vi "Force Sensing-Axial.vi"() -> ()   [LabVIEW 2010]
uses:
  <vilib>/Utility/file.llb/Write To Spreadsheet File (string).vi
panel:
  out "Shift 4":dbl
  out "Base 4":dbl format="%.3f"
  out "Channel 4":dbl format="%.2f"
  out "Calibration Constant":dbl
  in  "stop":bool
  in  "Force Scaling Factor":dbl=1.0
  in  "Record Switch":bool
  in  "file path (dialog if empty)":path=path "C:/Users/Berk/Desktop/closed_washer0_1"
  out "Measured Tip Forces [mN]":u8(slide) scale=0.0..10.0
  in  "Plot Switch":bool
  out "F [mN]":dbl format="%.1f"
  in  "sm130 IP Address":string="192.168.0.11"
  in  "Rebias":bool
  in  "Select Your Tool":T1(radio)
  out "Shift 3":dbl
  out "Shift 2":dbl
  out "Shift 1":dbl
  out "Channel 3":dbl format="%.2f"
  out "Channel 2":dbl format="%.2f"
  out "Channel 1":dbl format="%.2f"
  out "Base 3":dbl format="%.3f"
  out "Base 2":dbl format="%.3f"
  out "Base 1":dbl format="%.3f"
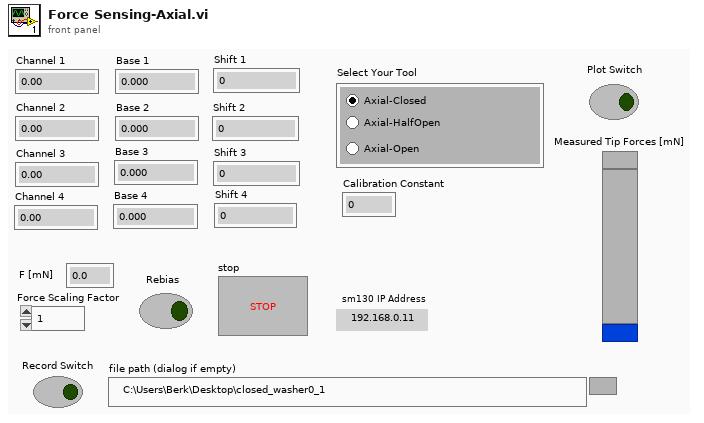
[diagram p1: front panel]
types:
  T1 = enum32{"Axial-Closed", "Axial-Open", "Axial-HalfOpen"}
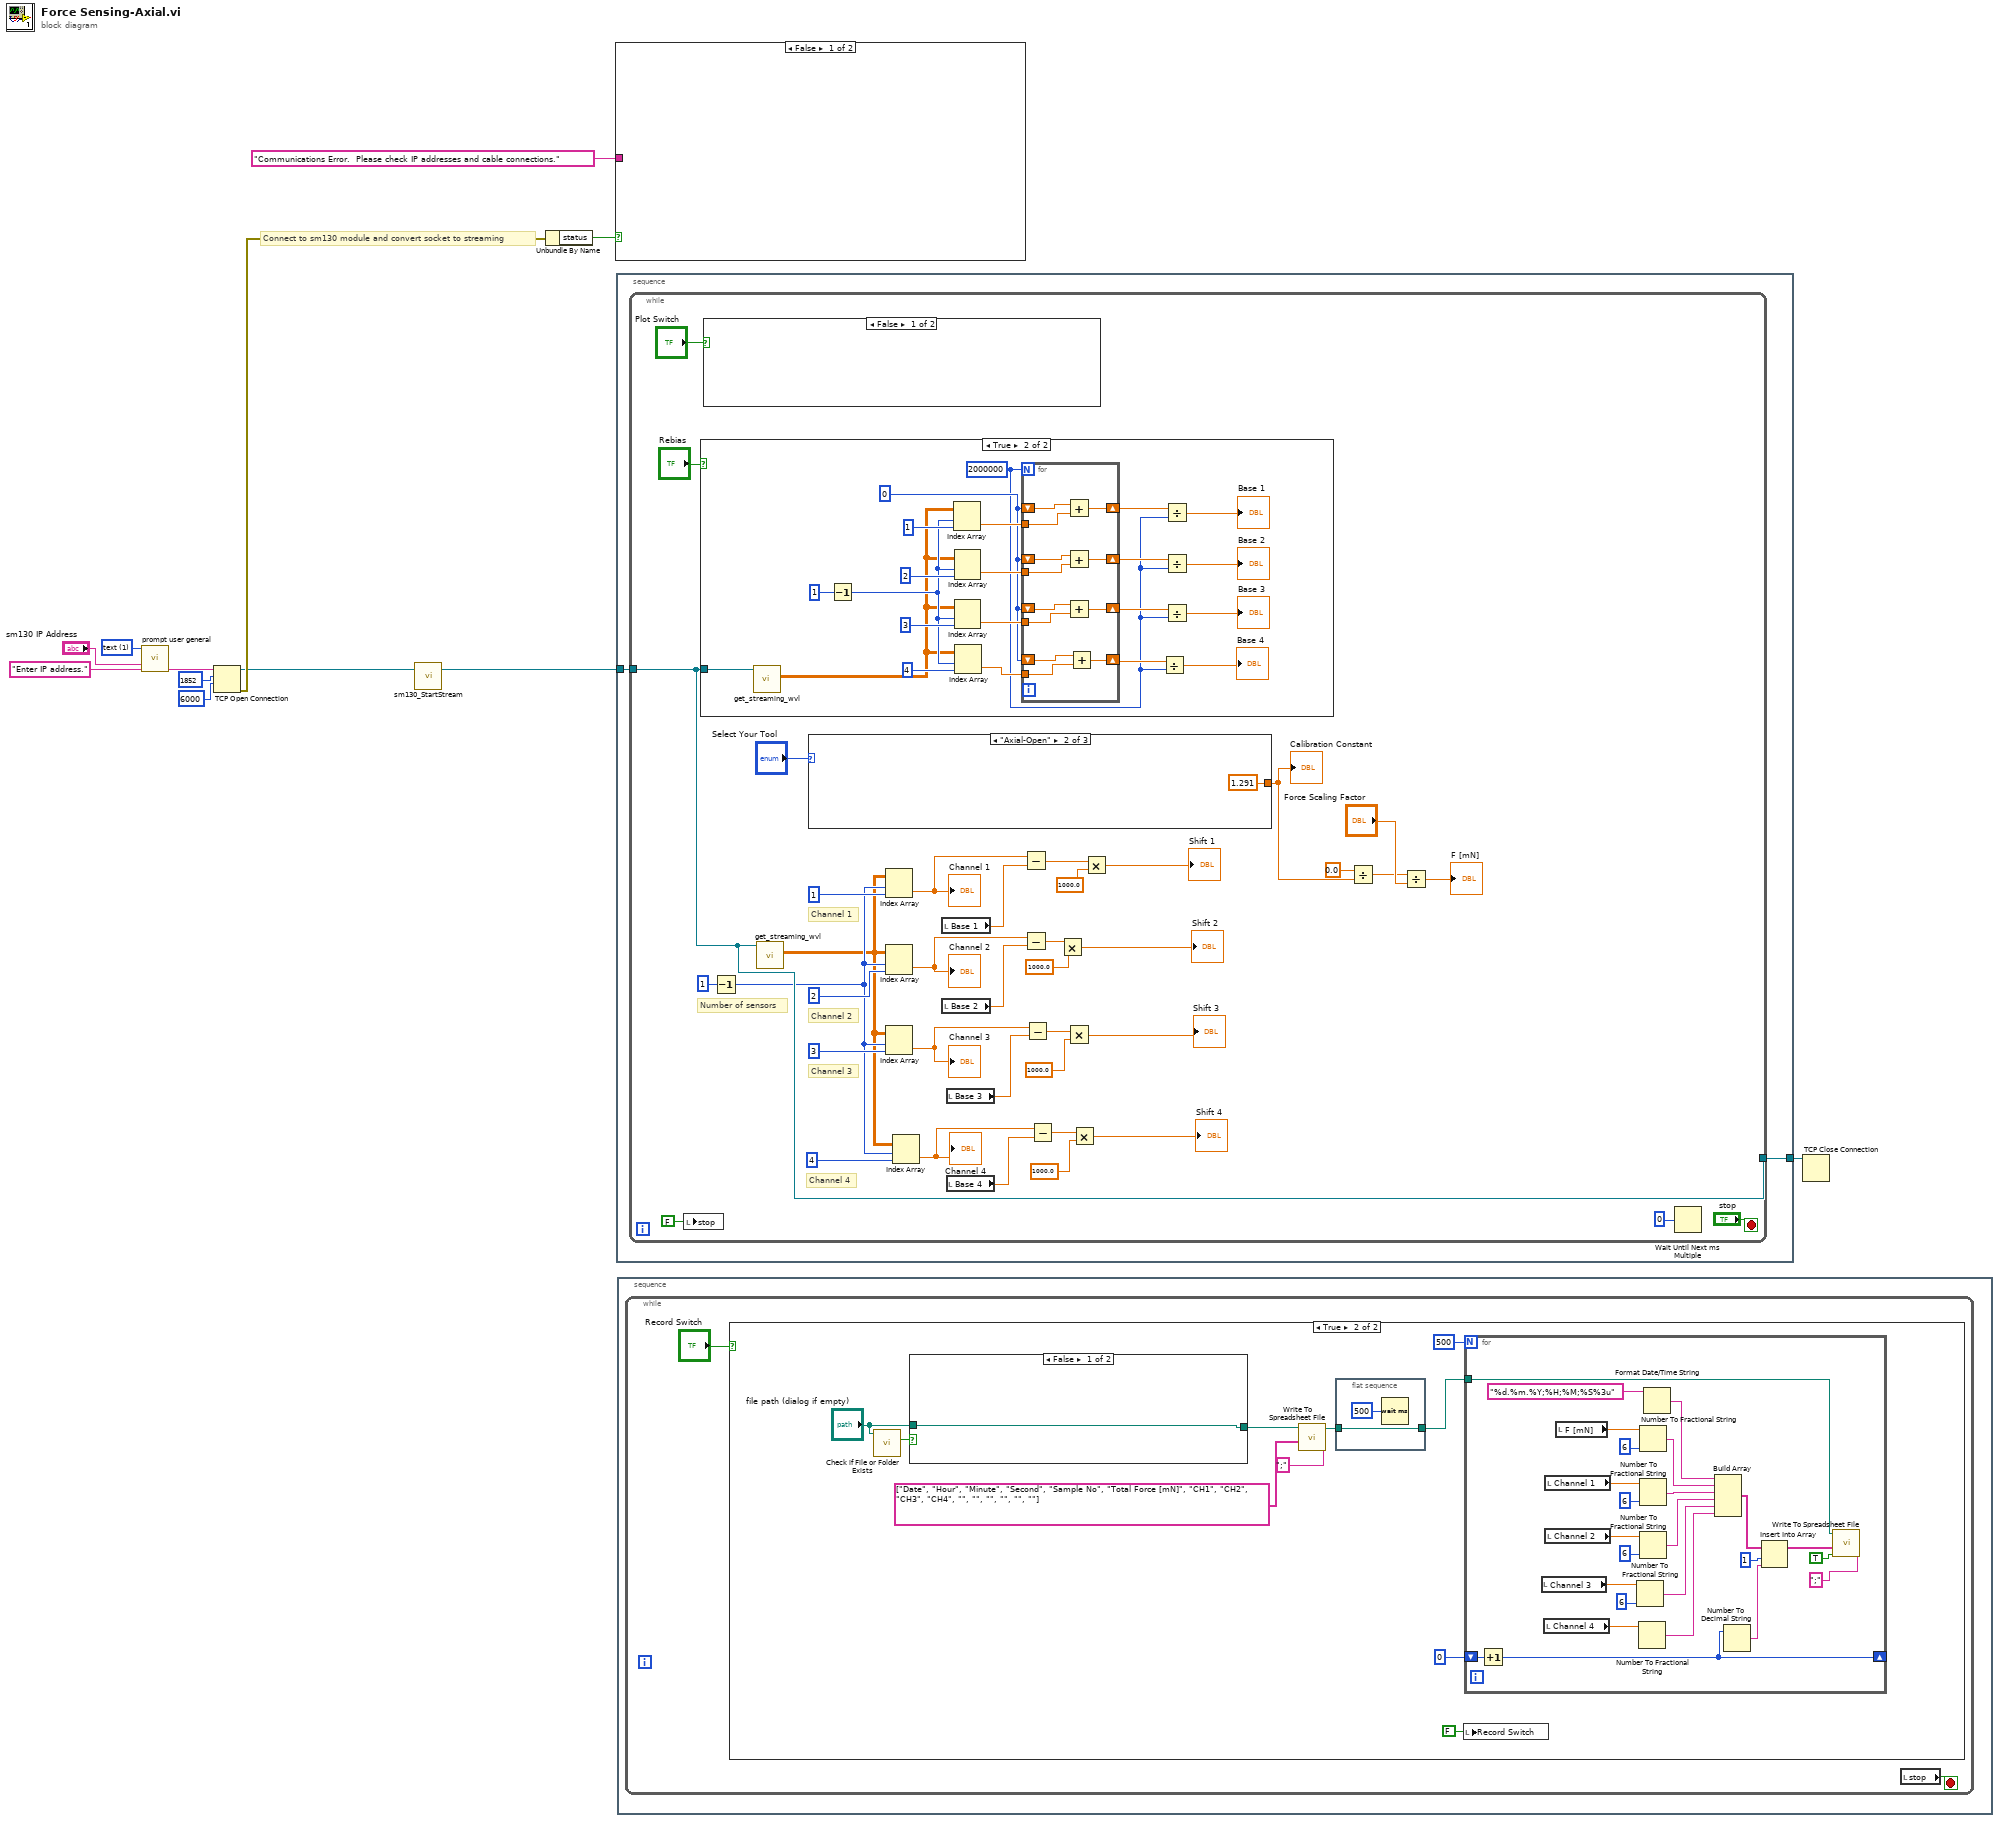
[diagram p0: block diagram]
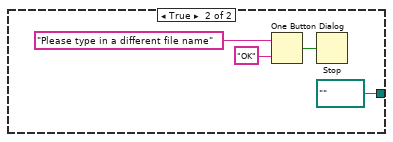
[diagram p3: hidden frame]
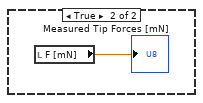
[diagram p4: hidden frame]
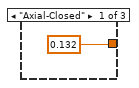
[diagram p6: hidden frame]
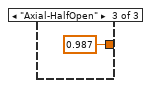
[diagram p7: hidden frame]
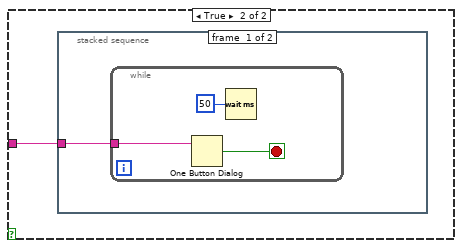
[diagram p8: hidden frame]
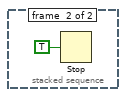
[diagram p9: hidden frame]
diagram:
  w9 = u16 1 items=["numeric", "text"] ("control type")
  # "Connect to sm130 module and convert socket to streaming"
  n1 = call "prompt user general.vi"("control type"=w9, "text default"="sm130 IP Address", "message to display"="Enter IP address.") -> ("Text output"=w4:string)  [unwired: 11 in, 1 out]
  n2 = TCP Open Connection(address=w4, remote port or service name=u16 1852 ("remote port"), timeout ms (60000)=6000) -> (connection ID=w1:refnum<k5>, error out=w6:errorcluster)  [unwired: 2 in]
  n3 = call "sm130_StartStream.vi"("Connection ID In"=w1) -> ("Stream ID Out"=w11:refnum<k5>)  [unwired: 1 in, 1 out]
  n4 = Unbundle By Name(w6) -> ("status"=w5:bool)
  n5 = case shown="False" w5 {
    tunnel: "Communications Error.  Please check IP addresses and cable connections." ("message") -> [_ w13]
    frame False {
    }
    frame True {
      n6 = stacked-sequence {
        tunnel: w13 -> [w14 _]
        frame #0 {
          n7 = while {
            tunnel: w14 -> [w15]
            stop <- w17 stop-if-true
            n8 = One Button Dialog(message=w15) -> (true=w17:bool)  [unwired: 1 in]
            n9 = Wait (ms)(milliseconds to wait=u32 50) -> ()  [unwired: 1 out]
          }
        }
        frame #1 {
          n10 = Stop(stop? (T)=TRUE) -> ()
        }
      }
    }
  }
  n11 = stacked-sequence {
    tunnel: w11 -> [w20]
    tunnel: [w19] -> w12
    frame #0 {
      n12 = while {
        tunnel: [w52] -> w19
        tunnel: w20 -> [w52]
        stop <- "stop" stop-if-true
        # "Channel 4"
        # "Channel 3"
        # "Channel 2"
        # "Channel 1"
        # "Number of sensors"
        n13 = local write "stop"(FALSE) -> ()
        n14 = case shown="True" "Rebias" {
          tunnel: w52 -> [_ w82]
          frame False {
          }
          frame True {
            w64 = 0
            w62 = 2000000
            n15 = call "get_streaming_wvl.vi"("Stream ID Out"=w82) -> ("Array"=w65:dbl[][])  [unwired: 9 in, 1 out]
            n16 = Decrement(x=1) -> (x-1=w70:i32)
            n17 = Index Array(array=w65, index (row)=w70, index (col)=1) -> (element=w75:dbl)
            n18 = Index Array(array=w65, index (row)=w70, index (col)=2) -> (element=w76:dbl)
            n19 = Index Array(array=w65, index (row)=w70, index (col)=3) -> (element=w77:dbl)
            n20 = Index Array(array=w65, index (row)=w70, index (col)=4) -> (element=w69:dbl)
            n21 = for {
              N: w62 -> [_]
              shift-right: [w88] -> w74
              shift-left: w64 -> [w87]
              shift-right: [w89] -> w73
              shift-left: w64 -> [w90]
              shift-right: [w94] -> w72
              shift-left: w64 -> [w92]
              tunnel: w77 -> [w93]
              tunnel: w76 -> [w91]
              tunnel: w75 -> [w86]
              shift-right: [w85] -> w63
              shift-left: w64 -> [w84]
              tunnel: w69 -> [w83]
              n22 = Add(x=w87, y=w86) -> (x+y=w88:dbl)
              n23 = Add(x=w90, y=w91) -> (x+y=w89:dbl)
              n24 = Add(x=w92, y=w93) -> (x+y=w94:dbl)
              n25 = Add(x=w84, y=w83) -> (x+y=w85:dbl)
            }
            n26 = Divide(x=w63, y=w62) -> (x/y=→"Base 4":dbl)
            n27 = Divide(x=w74, y=w62) -> (x/y=→"Base 1":dbl)
            n28 = Divide(x=w73, y=w62) -> (x/y=→"Base 2":dbl)
            n29 = Divide(x=w72, y=w62) -> (x/y=→"Base 3":dbl)
          }
        }
        n30 = case shown="False" "Plot Switch" {
          frame False {
          }
          frame True {
            n31 = local read "F [mN]"() -> (→"Measured Tip Forces [mN]":dbl)
          }
        }
        n32 = Decrement(x=1) -> (x-1=w31:i32)
        n33 = call "get_streaming_wvl.vi"("Stream ID Out"=w52) -> ("Array"=w30:dbl[][])  [unwired: 9 in, 1 out]
        n34 = case shown="\"Axial-Open\"" "Select Your Tool" {
          tunnel: [0.132 1.291 0.987] -> w36
          frame "Axial-Closed" {
          }
          frame "Axial-Open" {
          }
          frame "Axial-HalfOpen" {
          }
        }
        "Calibration Constant" <- w36
        n35 = Index Array(array=w30, index (row)=w31, index (col)=1) -> (element=w43:dbl)
        "Channel 1" <- w43
        n36 = Index Array(array=w30, index (row)=w31, index (col)=2) -> (element=w45:dbl)
        "Channel 2" <- w45
        n37 = Index Array(array=w30, index (row)=w31, index (col)=3) -> (element=w44:dbl)
        "Channel 3" <- w44
        n38 = Index Array(array=w30, index (row)=w31, index (col)=4) -> (element=w26:dbl)
        "Channel 4" <- w26
        n39 = local read "Base 1"() -> (w54:dbl)
        n40 = local read "Base 2"() -> (w53:dbl)
        n41 = local read "Base 3"() -> (w55:dbl)
        n42 = local read "Base 4"() -> (w25:dbl)
        n43 = Subtract(x=w43, y=w54) -> (x-y=w37:dbl)
        n44 = Subtract(x=w45, y=w53) -> (x-y=w38:dbl)
        n45 = Subtract(x=w44, y=w55) -> (x-y=w34:dbl)
        n46 = Subtract(x=w26, y=w25) -> (x-y=w28:dbl)
        n47 = Multiply(x=w38, y=1000.0) -> (x*y=→"Shift 2":dbl)
        n48 = Multiply(x=w34, y=1000.0) -> (x*y=→"Shift 3":dbl)
        n49 = Multiply(x=w28, y=1000.0) -> (x*y=→"Shift 4":dbl)
        n50 = Multiply(x=w37, y=1000.0) -> (x*y=→"Shift 1":dbl)
        n51 = Divide(x=0.0, y=w36) -> (x/y=w35:dbl)
        n52 = Divide(x=w35, y="Force Scaling Factor") -> (x/y=→"F [mN]":dbl)
        n53 = Wait Until Next ms Multiple(millisecond multiple=0) -> ()  [unwired: 1 out]
      }
    }
  }
  n54 = stacked-sequence {
    frame #0 {
      n55 = while {
        stop <- w98 stop-if-true
        n56 = case shown="True" "Record Switch" {
          frame False {
          }
          frame True {
            n57 = call <vilib>:"Check if File or Folder Exists.vi"("path"="file path (dialog if empty)") -> ("file or folder exists?"=w106:bool)  [unwired: 8 in, 2 out]
            n58 = case shown="False" w106 {
              tunnel: [w135 path "" ("file path (dialog if empty)")] -> w107
              tunnel: "file path (dialog if empty)" -> [w135 _]
              frame False {
              }
              frame True {
                n59 = One Button Dialog(message="Please type in a different file name", button name ("OK")="OK") -> (true=w137:bool)
                n60 = Stop(stop? (T)=w137) -> ()
              }
            }
            n61 = call-poly <vilib>:"Write To Spreadsheet File.vi"("delimiter (\\t)"=";" ("delimiter (\\t)"), "1D data"=string[] ["Date", "Hour", "Minute", "Second", "Sample No", "Total Force [mN]", "CH1", "CH2", "CH3", "CH4", "", "", "", "", "", ""], "file path (dialog if empty)"=w107) -> ("new file path (Not A Path if cancelled)"=w104:path)  [unwired: 5 in]
            n62 = flat-sequence {
              tunnel: [w140] -> w103
              tunnel: w104 -> [w140]
              frame #0 {
                n63 = Wait (ms)(milliseconds to wait=u32 500) -> ()  [unwired: 1 out]
              }
            }
            n64 = local write "Record Switch"(FALSE ("Record Switch")) -> ()
            n65 = for {
              N: 500 -> [_]
              shift-right: [w130] -> _
              shift-left: 0 -> [w123]
              tunnel: w103 -> [w122]
              n66 = Increment(x=w123) -> (x+1=w130:i32)
              n67 = local read "Channel 3"() -> (w114:dbl)
              n68 = local read "Channel 4"() -> (w112:dbl)
              n69 = local read "Channel 1"() -> (w118:dbl)
              n70 = local read "Channel 2"() -> (w119:dbl)
              n71 = local read "F [mN]"() -> (w125:dbl)
              n72 = Number To Fractional String(number=w114, precision (6)=i16 6) -> (F-format string=w111:string)  [unwired: 2 in]
              n73 = Number To Fractional String(number=w112) -> (F-format string=w110:string)  [unwired: 3 in]
              n74 = Number To Fractional String(number=w125, precision (6)=i16 6) -> (F-format string=w124:string)  [unwired: 2 in]
              n75 = Number To Fractional String(number=w118, precision (6)=i16 6) -> (F-format string=w116:string)  [unwired: 2 in]
              n76 = Number To Fractional String(number=w119, precision (6)=i16 6) -> (F-format string=w115:string)  [unwired: 2 in]
              n77 = Format Date/Time String(time format string (%c)="%d.%m.%Y;%H;%M;%S%3u") -> (date/time string=w117:string)  [unwired: 2 in]
              n78 = Build Array(w117, w124, w116, w115, w111, w110) -> (w133:string[])
              n79 = Number To Decimal String(number=w130) -> (decimal integer string=w131:string)  [unwired: 1 in]
              n80 = Insert Into Array(array=w133, index=1, new element=w131) -> (w129:string[])
              n81 = call-poly <vilib>:"Write To Spreadsheet File.vi"("delimiter (\\t)"=";" ("delimiter (\\t)"), "append to file? (new file:F)"=TRUE, "1D data"=w129, "file path (dialog if empty)"=w122) -> ()  [unwired: 4 in, 1 out]
            }
          }
        }
        n82 = local read "stop"() -> (w98:bool)
      }
    }
  }
  n83 = TCP Close Connection(connection ID=w12) -> ()  [unwired: 2 in, 2 out]
